vi "CHD_DRIVE_BEGIN.vi"(8 "error in (no error)":errorcluster) -> (0 "error out":errorcluster, 2 "Gyro Reading":T1 {"SIN" format="%13.4f"; "COS" format="%13.4f"; "VALUE" format="%13.4f"}, 3 "DIFF_DRIVE_KINEMATICS":T2 {"TrackWidth_Meters" format="%20.4f"})   [LabVIEW 2019]
uses:
  <vilib>/Rock Robotics/WPI/ThirdParty/JAS_Junk/TrajLib/TypeDef/DIFF_DRIVE_KINEMATICS.ctl
  <vilib>/Rock Robotics/WPI/ThirdParty/JAS_Junk/TrajLib/TypeDef/ROTATION2D.ctl
  <vilib>/Rock Robotics/SystemInterfaces/DIO/FPGA_DIOPWMChannel.ctl
  <vilib>/Rock Robotics/SystemInterfaces/DIO/FPGA_DIOChannel.ctl
  <vilib>/Rock Robotics/SystemInterfaces/AI/FPGA_AIGyroChannel.ctl
  <vilib>/Rock Robotics/SystemInterfaces/NetworkCommunication/NetComm_UsageReport_report.vi
  <vilib>/Rock Robotics/WPI/ThirdParty/JAS_Junk/TrajLib/VI/BoolCmd_Send_Internal.vi
  <vilib>/Rock Robotics/WPI/ThirdParty/JAS_Junk/TrajLib/Conv_Deg_Radians.vi
  <vilib>/Rock Robotics/WPI/ThirdParty/JAS_Junk/TrajLib/Rotation2d_CreateAngle.vi
  <vilib>/Rock Robotics/WPI/ThirdParty/JAS_Junk/TrajLib/VI/BoolCmd_ObtainQueue.vi
  <vilib>/Rock Robotics/WPI/ThirdParty/JAS_Junk/TrajLib/Globals/Util_LibraryGlobals.vi
  CHD_DRIVE_GLOBALS.vi
  <vilib>/Rock Robotics/WPI/ThirdParty/JAS_Junk/TrajLib/Trajectory_Library.lvlib
  <vilib>/Rock Robotics/WPI/Gyro/WPI_GyroAnalogOpen.vi
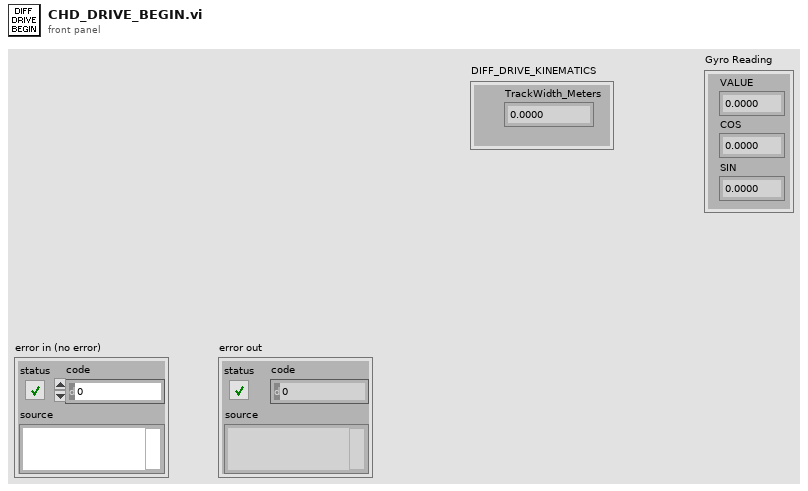
[diagram p1: front panel]
types:
  T1 = typedef "Trajectory_Library.lvlib/ROTATION2D.ctl" = cluster{"VALUE":dbl, "COS":dbl, "SIN":dbl}
  T2 = typedef "Trajectory_Library.lvlib/DIFF_DRIVE_KINEMATICS.ctl" = cluster{"TrackWidth_Meters":dbl}
  T3 = typedef "FPGA_AIGyroChannel.ctl" = enum8{"AI 0", "AI 1", "Invalid"}
  T4 = typedef "FPGA_DIOChannel.ctl" = enum8{"DIO 0", "DIO 1", "DIO 2", "DIO 3", "DIO 4", "DIO 5", "DIO 6", "DIO 7", "DIO 8", "DIO 9", "DIO MXP 0", "DIO MXP 1", "DIO MXP 2", "DIO MXP 3", "DIO MXP 4", "DIO MXP 5", "DIO MXP 6", "DIO MXP 7", "DIO MXP 8", "DIO MXP 9", "DIO MXP 10", "DIO MXP 11", "DIO MXP 12", "DIO MXP 13", "DIO MXP 14", "DIO MXP 15", "SPI Port CS1", "SPI Port CS2", "SPI Port CS3", "SPI Port MISO", "SPI Port MOSI", "Invalid"}
  T5 = typedef "FPGA_DIOPWMChannel.ctl" = enum8{"PWM 0", "PWM 1", "PWM 2", "PWM 3", "PWM 4", "PWM 5", "PWM 6", "PWM 7", "PWM 8", "PWM 9", "PWM MXP 0", "PWM MXP 1", "PWM MXP 2", "PWM MXP 3", "PWM MXP 4", "PWM MXP 5", "PWM MXP 6", "PWM MXP 7", "PWM MXP 8", "PWM MXP 9", "Invalid"}
  T6 = typedef "WPI_GyroDevRef.ctl" = cluster{"DevStatus":errorcluster, "Analog Channel":T7, "Gain (VoltsPerDegree/Second)":dbl, "Gyro Type":enum16{"Analog", "XRS450"}, "Handle":i32, "SPI Bus":T8, "Device Found":bool, "Sample Rate":dbl, "Calibrate On Open":bool, "Offset":dbl}
  T7 = typedef "FPGA_AIChannel.ctl" = enum8{"AI 0", "AI 1", "AI 2", "AI 3", "AI MXP 0", "AI MXP 1", "AI MXP 2", "AI MXP 3", "Invalid"}
  T8 = typedef "spi_bus.ctl" = enum16{"SPI On-Board, CS0", "SPI On-Board, CS1", "SPI On-Board, CS2", "SPI On-Board, CS3", "SPI MXP", "Invalid"}
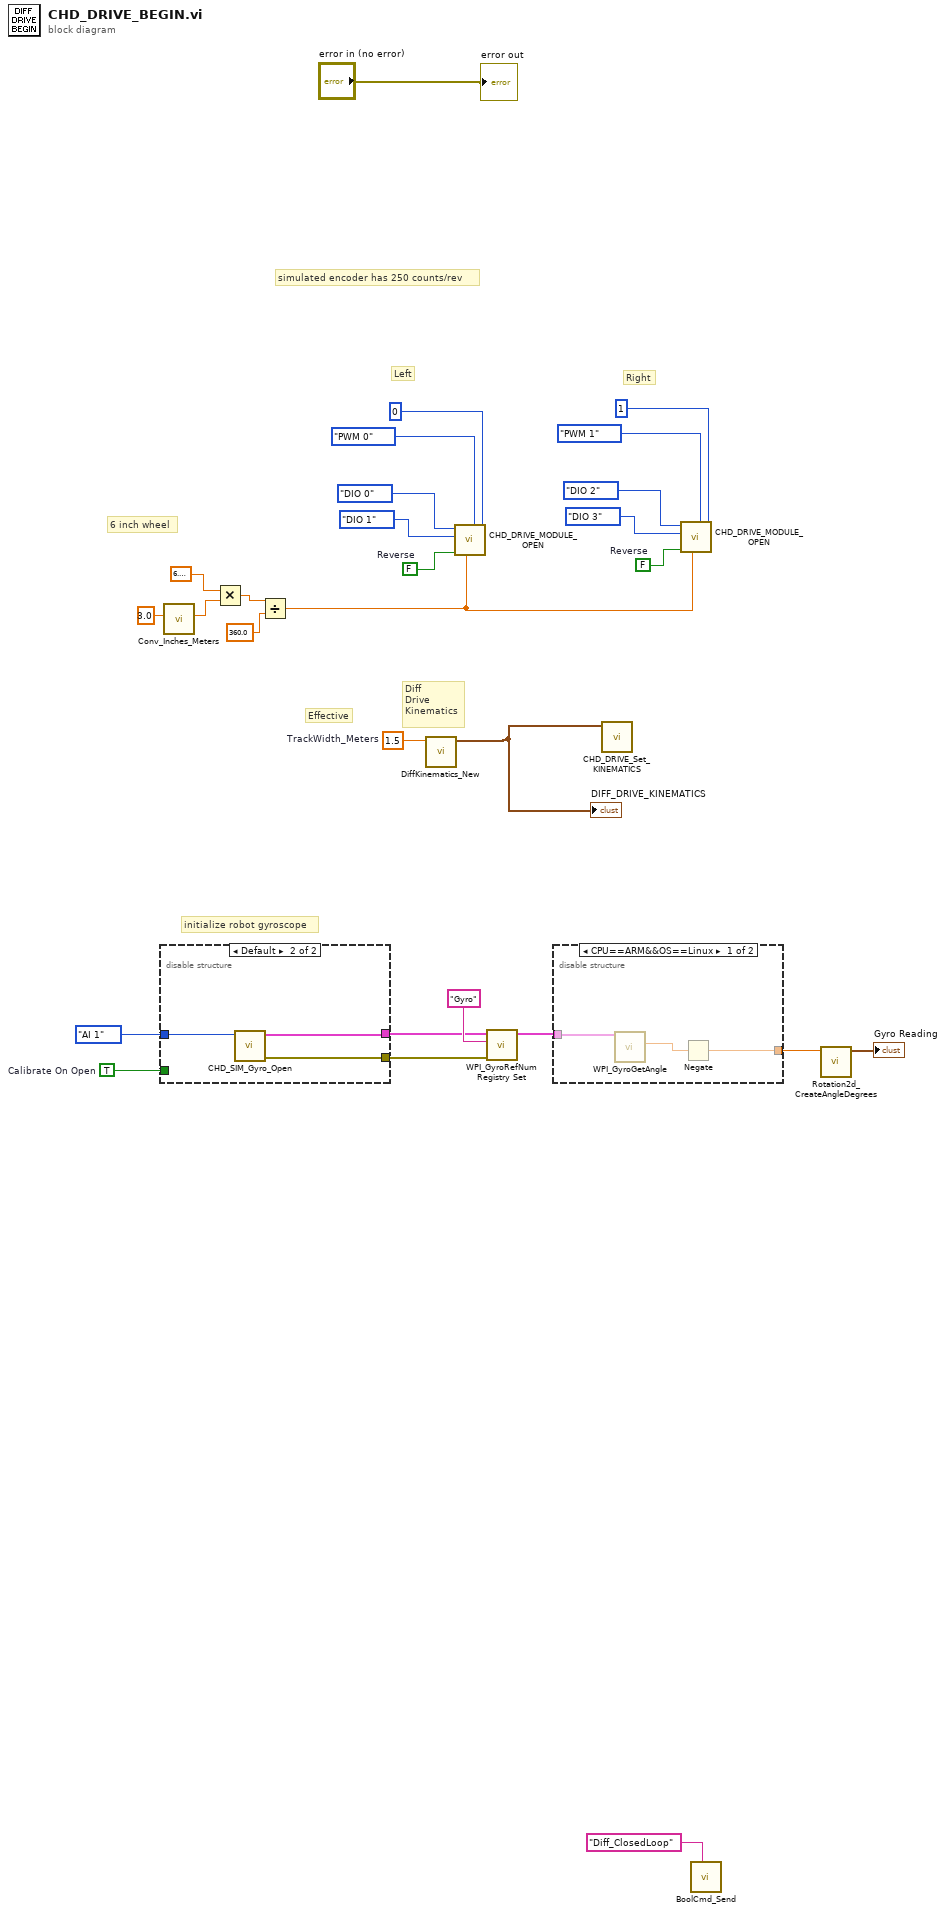
[diagram p0: block diagram]
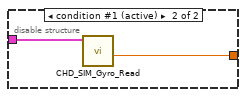
[diagram p2: hidden frame]
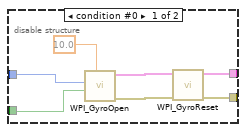
[diagram p3: hidden frame]
diagram:
  w1 = FALSE  # Reverse
  w2 = FALSE  # Reverse
  w4 = 1.5  # TrackWidth_Meters
  w12 = TRUE  # Calibrate On Open
  # "Right"
  # "Left"
  # "Effective"
  # "Diff\nDrive\nKinematics"
  # "6 inch wheel"
  # "initialize robot gyroscope"
  # "simulated encoder has 250 counts/rev"
  n1 = disable-structure shown="Default" {
    disable-tunnel: w12 -> [w32 _]
    disable-tunnel: [w31 w38] -> w11
    disable-tunnel: [w30 w37] -> w10
    disable-tunnel: FPGA_AIGyroChannel."AI 1" ("Analog Channel") -> [w29 w36]
    frame condition #0 {
      n2 = call-poly <vilib>:"WPI_GyroOpen.vi"("Calibration Time (s)"=10.0, "Calibrate On Open"=w32, "Analog Channel"=w29) -> ("error out"=w33:errorcluster, "GyroDevRef"=w34:T6)  [unwired: 6 in, 1 out]
      n3 = call <vilib>:"WPI_GyroReset.vi"("error in (no error)"=w33, "GyroDevRef"=w34) -> ("error out"=w30:errorcluster, "GyroDevRef"=w31:T6)  [unwired: 8 in]
    }
    frame condition #1 (active) {
      n4 = call "CHD_SIM_Gyro_Open.vi"("Analog Channel"=w36) -> ("error out"=w37:errorcluster, "GyroDevRef"=w38:T6)  [unwired: 9 in]
    }
  }
  n5 = call <vilib>:"Conv_Inches_Meters.vi"("INCH"=3.0) -> ("Meters"=w26:dbl)  [unwired: 10 in]
  n6 = Multiply(x=6.283185307179586, y=w26) -> (x*y=w14:dbl)
  n7 = Divide(x=w14, y=360.0) -> (x/y=w28:dbl)
  n8 = call <vilib>:"DiffKinematics_New.vi"("TrackWidth_Meters"=w4) -> ("DIFF_DRIVE_KINEMATICS"=w3:T2)  [unwired: 10 in]
  "DIFF_DRIVE_KINEMATICS" <- w3
  n9 = call "CHD_DRIVE_MODULE_OPEN.vi"("Module Index"=0 ("NameSuffix"), "Drive PWM Channel"=FPGA_DIOPWMChannel."PWM 0", "DistancePerCount"=w28, "Reverse"=w2, "Drive B Channel"=FPGA_DIOChannel."DIO 1", "Drive A channel"=FPGA_DIOChannel."DIO 0") -> ()  [unwired: 6 in]
  n10 = call <vilib>:"WPI_GyroRefNum Registry Set.vi"("error in (no error)"=w10, "refnum name"="Gyro", "GyroDevRef"=w11) -> ("GyroDevRef"=w8:T6)  [unwired: 7 in, 1 out]
  n11 = disable-structure shown="CPU==ARM&&OS==Linux" {
    disable-tunnel: w8 -> [w41 w43]
    disable-tunnel: [w39 w42] -> w7
    frame condition #0 {
      n12 = call <vilib>:"WPI_GyroGetAngle.vi"("GyroDevRef"=w41) -> ("Angle"=w40:dbl)  [unwired: 6 in, 4 out]
      n13 = Negate(x=w40) -> (-x=w39:dbl)
    }
    frame condition #1 (active) {
      n14 = call "CHD_SIM_Gyro_Read.vi"("GyroDevRef"=w43) -> ("Gyro_Cont_Deg"=w42:dbl)  [unwired: 10 in]
    }
  }
  n15 = call "CHD_DRIVE_Set_KINEMATICS.vi"("DIFF_DRIVE_KINEMATICS"=w3) -> ()  [unwired: 11 in]
  n16 = call "CHD_DRIVE_MODULE_OPEN.vi"("Module Index"=1 ("NameSuffix"), "Drive PWM Channel"=FPGA_DIOPWMChannel."PWM 1", "DistancePerCount"=w28, "Reverse"=w1, "Drive B Channel"=FPGA_DIOChannel."DIO 3", "Drive A channel"=FPGA_DIOChannel."DIO 2") -> ()  [unwired: 6 in]
  n17 = call <vilib>:"BoolCmd_Send.vi"("Command Name"="Diff_ClosedLoop") -> ()  [unwired: 10 in, 1 out]
  n18 = call <vilib>:"Rotation2d_CreateAngleDegrees.vi"("Angle_Degrees"=w7) -> ("ROTATION"=→"Gyro Reading":T1)  [unwired: 10 in]
  "error out" <- "error in (no error)"
